vi "Phase Extraction.vi"(1 "Array 2":dbl[](array[numeric])) -> (0 "detected phase (deg)":dbl format="%.2p", 2 "Regenerated phase wrapped":dbl[](graph), 3 "Envelope":dbl[](graph), 4 "detected frequency":dbl format="%.4p", 5 "Normalized Envelope":waveform(dbl)(graph), 6 "Array":dbl[](array[numeric]))   [LabVIEW 2009]
uses:
  <vilib>/measure/matone.llb/Extract Single Tone Information 1 Chan.vi
  <vilib>/Analysis/3filter.llb/Butterworth Filter (DBL).vi
  <vilib>/Analysis/NI_AALBase.lvlib
  <vilib>/measure/NI_MAPro.lvlib
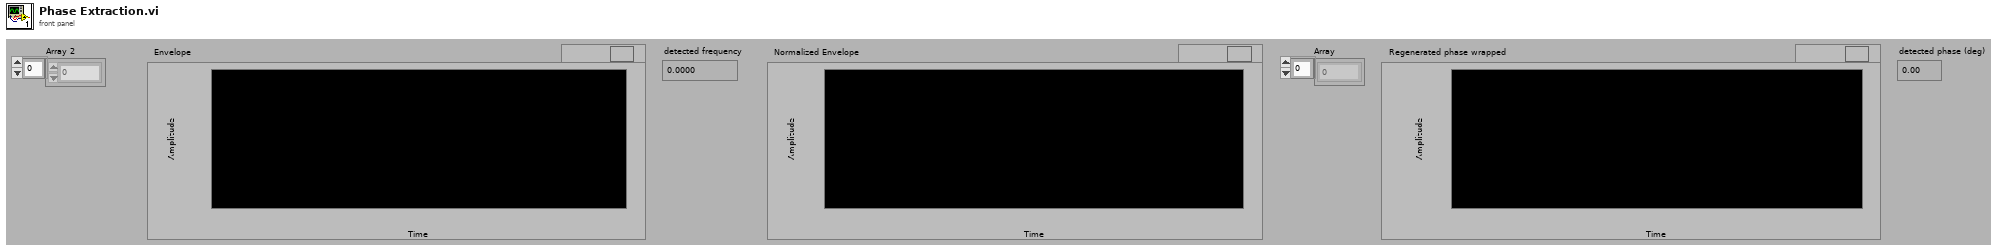
[diagram p1: front panel]
types:
  T1 = enum32{"Lowpass", "Highpass", "Bandpass", "Bandstop"}
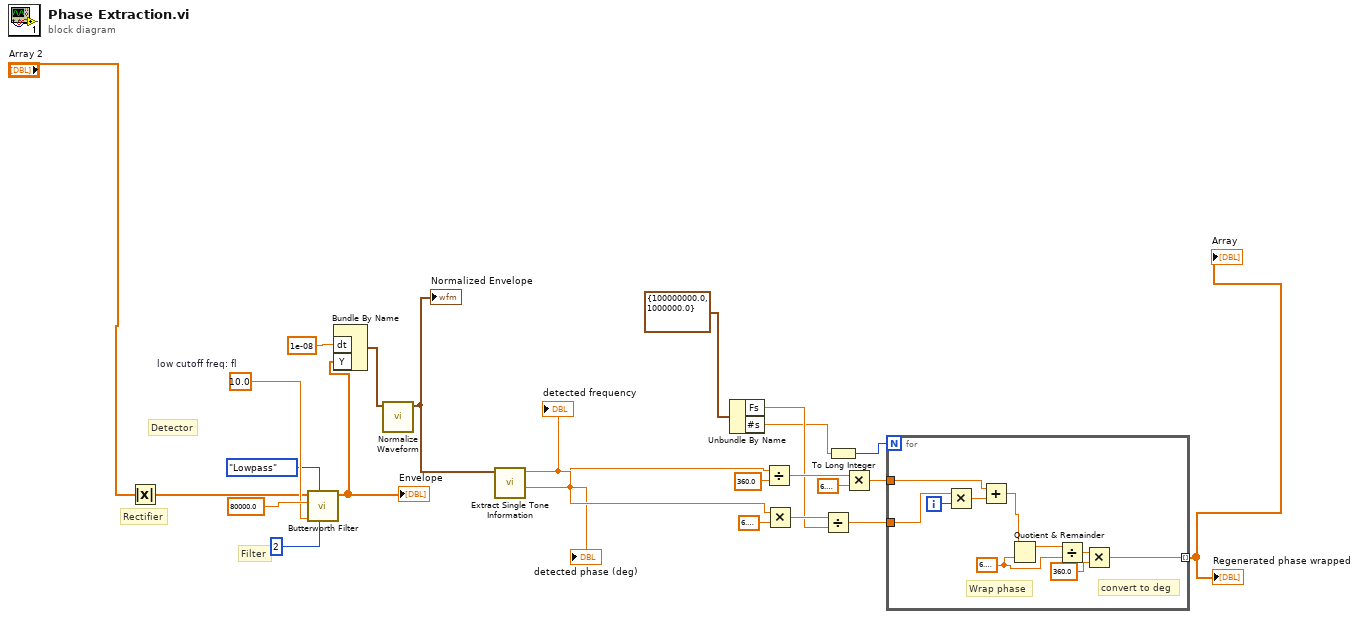
[diagram p0: block diagram]
diagram:
  w3 = 10.0  # low cutoff freq: fl
  # "Detector"
  # "Filter"
  # "Rectifier"
  n1 = Absolute Value(x="Array 2") -> (abs(x)=w2:dbl[])
  n2 = call-poly <vilib>:"Butterworth Filter.vi"("order"=2, "filter type"=T1."Lowpass", "low cutoff freq: fl"=w3, "sampling freq: fs"=80000.0, "X"=w2) -> ("Filtered X"=w22:dbl[])  [unwired: 3 in, 1 out]
  "Envelope" <- w22
  n3 = Bundle By Name("dt"=1e-08, "Y"=w22) -> (w7:waveform(dbl))  [unwired: 1 in]
  n4 = call <vilib>:"Normalize Waveform.vi"("waveform in"=w7) -> ("normalized waveform"=w8:waveform(dbl))  [unwired: 7 in, 3 out]
  "Normalized Envelope" <- w8
  n5 = call-poly <vilib>:"Extract Single Tone Information.vi"("time signal in"=w8) -> ("detected phase (deg)"=w20:dbl, "detected frequency"=w21:dbl)  [unwired: 5 in, 4 out]
  "detected frequency" <- w21
  "detected phase (deg)" <- w20
  n6 = Unbundle By Name(cluster{"Fs":dbl, "#s":dbl} {"Fs"=100000000.0, "#s"=1000000.0} ("sampling info")) -> ("Fs"=w11:dbl, "#s"=w10:dbl)
  n7 = Divide(x=w20, y=360.0) -> (x/y=w17:dbl)
  n8 = Multiply(x=w21, y=6.283185307179586) -> (x*y=w14:dbl)
  n9 = Divide(x=w14, y=w11) -> (x/y=w13:dbl)
  n10 = To Long Integer(number=w10) -> (32bit integer=w9:i32)
  n11 = Multiply(x=w17, y=6.283185307179586) -> (x*y=w12:dbl)
  n12 = for {
    N: w9 -> [_]
    tunnel: w13 -> [w33]
    tunnel: w12 -> [w32]
    tunnel: [w27] -> w24 mode=indexing
    i -> [w34]
    w30 = 6.283185307179586
    # "convert to deg"
    # "Wrap phase"
    n13 = Multiply(x=w33, y=w34) -> (x*y=w31:dbl)
    n14 = Add(x=w32, y=w31) -> (x+y=w26:dbl)
    n15 = Quotient & Remainder(x=w26, y=w30) -> (x-y*floor(x/y)=w25:dbl)  [unwired: 1 out]
    n16 = Divide(x=w25, y=w30) -> (x/y=w29:dbl)
    n17 = Multiply(x=w29, y=360.0) -> (x*y=w27:dbl)
  }
  "Regenerated phase wrapped" <- w24
  "Array" <- w24
